vi "sum.vi"(8 "error in (no error)":errorcluster, 10 "b":i32, 11 "a":i32) -> (0 "error out":errorcluster, 3 "function return":i32)   [LabVIEW 2021, in "new_libmath.lvlib"]
doc: "int sum(int a, int b);"
uses:
  <userlib>/new_libmath/new_libmath.lvlib
  <userlib>/new_libmath/libmath.dll
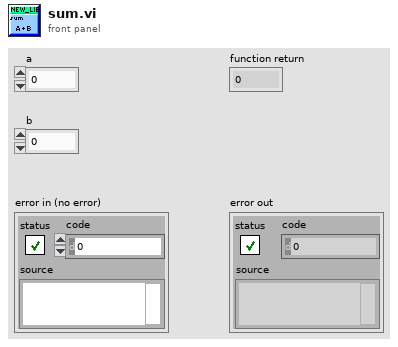
[diagram p1: front panel]
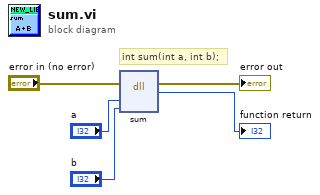
[diagram p0: block diagram]
diagram:
  # "int sum(int a, int b);"
  n1 = dll-call lib="C:/Program Files (x86)/National Instruments/LabVIEW 2021/user.lib/new_libmath/libmath.*" fn="sum"(error in="error in (no error)", "a"="a", "b"="b") -> (error out=→"error out":errorcluster, →"function return":i32)  [unwired: 4 in, 1 out]
